vi "Access insert values.vi"(5 "是否创建唯一键":bool, 6 "Password":string, 7 "data":variant[](array[variant]), 8 "error in (no error)":errorcluster, 9 "columns外部输入":T1, 10 "database":string="database1.mdb", 11 "table":string) -> (0 "error out":errorcluster)   [LabVIEW 2016, in "Access Lib.lvlib"]
uses:
  Access Lib.lvlib
  <vilib>/addons/database/Auxilliary.llb/DB Tools Transaction.ctl
  <vilib>/addons/database/Auxilliary.llb/DB Tools Isolation Level.ctl
  <vilib>/addons/database/Auxilliary.llb/DB Tools Column Info.ctl
  <vilib>/addons/database/Auxilliary.llb/DB Tools DataTypes.ctl
  <vilib>/addons/database/Auxilliary.llb/DB Tools Parameter Info.ctl
  <vilib>/addons/database/Auxilliary.llb/DB Tools Parameter Dir.ctl
  <vilib>/addons/database/Connection.llb/DB Tools Open Connec (String).vi
  <vilib>/addons/database/Connection.llb/Conn Transaction.vi
  <vilib>/addons/database/Connection.llb/Conn Execute.vi
  <vilib>/addons/database/Recordset.llb/Rec Destroy - Connection.vi
  <vilib>/addons/database/Command.llb/Cmd Set Parameter Value (C).vi
  <vilib>/addons/database/Command.llb/Cmd Execute.vi
  <vilib>/addons/database/Recordset.llb/Rec Destroy - Command.vi
  <vilib>/addons/database/Command.llb/Cmd Delete.vi
  <vilib>/addons/database/NI_Database_API.lvlib
  <vilib>/Utility/VariantDataType/VariantType.lvlib
panel:
  out "当前数据时间":timestamp
  out "当前测量模式":string
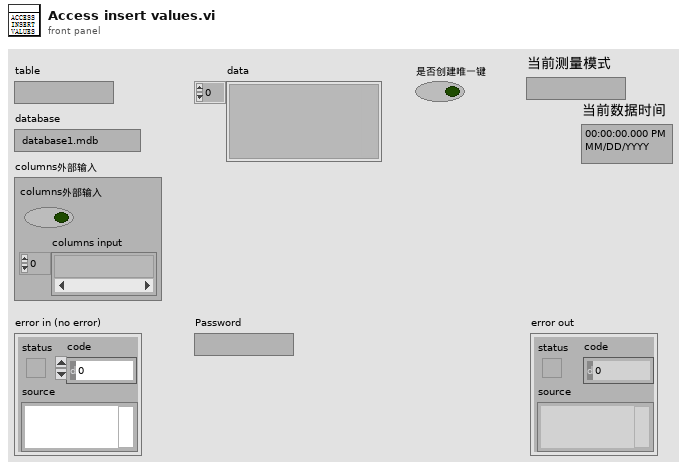
[diagram p1: front panel]
types:
  T1 = cluster{"columns外部输入":bool, "columns input":string[]}
  T2 = typedef "NI_Database_API.lvlib/DB Tools Isolation Level.ctl" = enum16{"chaos", "read uncommitted", "read committed", "repeatable read", "serializable"}
  T3 = typedef "NI_Database_API.lvlib/DB Tools Transaction.ctl" = enum16{"begin", "commit", "rollback"}
  T4 = typedef "NI_Database_API.lvlib/DB Tools Column Info.ctl" = cluster{"column name":string, "data type":T5, "size":i32, "allow null?":bool}
  T5 = typedef "NI_Database_API.lvlib/DB Tools DataTypes.ctl" = enum16{"String", "Long (I32)", "Single (SGL)", "Double (DBL)", "Date/Time", "Binary"}
  T6 = typedef "VariantType.lvlib/Type.ctl" = enum8{"Invalid Type", "Void", "I8", "I16", "I32", "I64", "U8", "U16", "U32", "U64", "Single Float", "Double Float", "Extended Float", "Single Complex", "Double Complex", "Extended Complex", "Enum U8", "Enum U16", "Enum U32", "Enum U64", "Single Float With Unit", "Double Float With Unit", "Extended Float With Unit", "Single Complex with Unit", "Double Complex with Unit", "Extended Complex with Unit", "Boolean", "String", "Path", "Picture", "Tag", "Array", "Cluster", "Variant", "LV Variant", "Waveform", "Timestamp", "Digital Waveform", "Digital Data", "ExpressData", "Refnum", "External Data", "VI", "Poly VI", "LabVIEW Class Instance", "Fixed Point"}
  T7 = typedef "NI_Database_API.lvlib/Conn ObjectReference.ctl" = refnum<k1>
  T8 = typedef "NI_Database_API.lvlib/DB Tools Parameter Info.ctl" = cluster{"parameter name":string, "type":T5, "direction":T9, "value":variant}
  T9 = typedef "NI_Database_API.lvlib/DB Tools Parameter Dir.ctl" = enum32{"Input", "Output", "Input/Output", "Return Value"}
  T10 = typedef "NI_Database_API.lvlib/Rec ObjectReference.ctl" = refnum<k1>
  T11 = typedef "LVDateTimeRec.ctl" = cluster{"秒数的小数部分":dbl, "秒":i32, "分":i32, "时":i32, "日":i32, "月":i32, "年":i32, "天数（周）":i32, "天数（年）":i32, "DST":i32}
  T12 = typedef "NI_Database_API.lvlib/Cmd ObjectReference.ctl" = refnum<k1>
  T13 = typedef "NI_Database_API.lvlib/Cmd-Rec Object Reference.ctl" = refnum<k1>
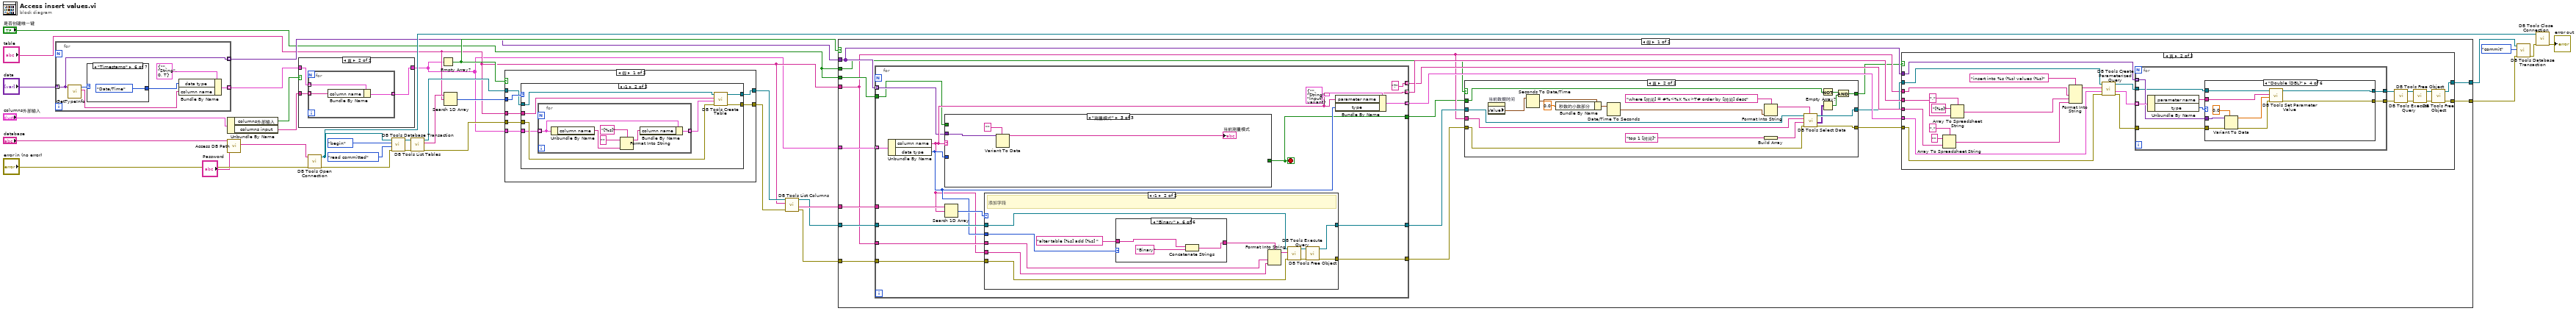
[diagram p0: block diagram]
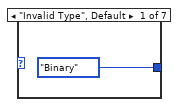
[diagram p3: hidden frame]
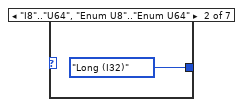
[diagram p4: hidden frame]
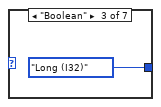
[diagram p5: hidden frame]
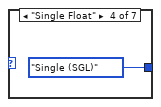
[diagram p6: hidden frame]
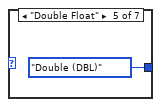
[diagram p7: hidden frame]
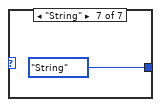
[diagram p8: hidden frame]
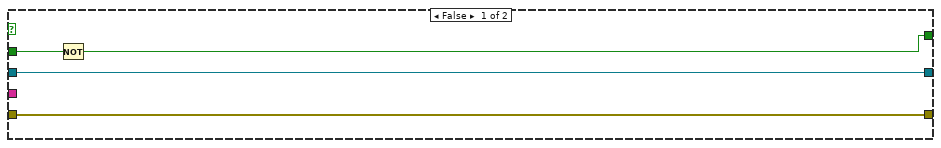
[diagram p11: hidden frame]
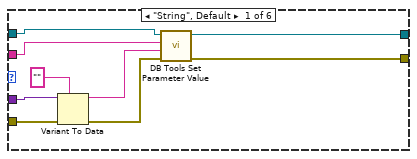
[diagram p13: hidden frame]
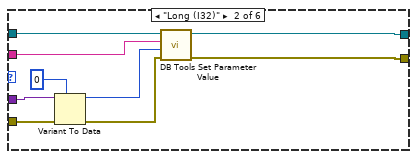
[diagram p14: hidden frame]
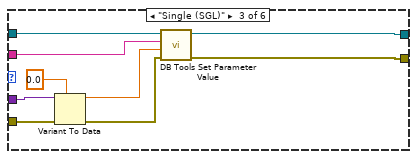
[diagram p15: hidden frame]
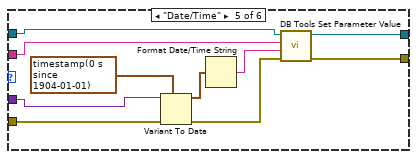
[diagram p16: hidden frame]
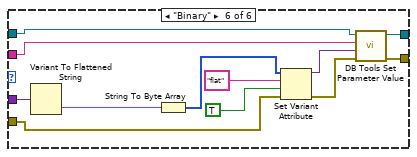
[diagram p17: hidden frame]
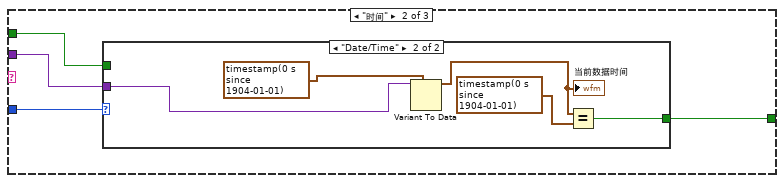
[diagram p19: hidden frame]
diagram:
  n1 = for {
    tunnel: [w35] -> w12 mode=indexing
    tunnel: [w37] -> w9 mode=indexing
    tunnel: "data" -> [w35] mode=indexing
    n2 = call <vilib>:"GetTypeInfo.vi"("Variant"=w35) -> ("Name"=w36:string, "Type Enum"=w39:T6)  [unwired: 6 in, 3 out]
    n3 = case shown="\"Timestamp\"" w39 {
      tunnel: [DB_Tools_DataTypes."Binary" ("data type") DB_Tools_DataTypes."Long (I32)" ("data type") DB_Tools_DataTypes."Long (I32)" ("data type") DB_Tools_DataTypes."Single (SGL)" ("data type") DB_Tools_DataTypes."Double (DBL)" ("data type") DB_Tools_DataTypes."Date/Time" ("data type") DB_Tools_DataTypes."String" ("data type")] -> w38
      frame "Invalid Type", Default {
      }
      frame "I8".."U64", "Enum U8".."Enum U64" {
      }
      frame "Boolean" {
      }
      frame "Single Float" {
      }
      frame "Double Float" {
      }
      frame "Timestamp" {
      }
      frame "String" {
      }
    }
    n4 = Bundle By Name(cluster=T4 {"column name"="", "data type"=enum."String", "size"=0, "allow null?"=TRUE} ("column information"), "data type"=w38, "column name"=w36) -> (w37:T4)
  }
  n5 = Unbundle By Name("columns外部输入") -> ("columns外部输入"=w7:bool, "columns input"=w8:string[])
  n6 = call "Access DB Path.vi"("Password"="Password", "database"="database") -> ("Connection information"=w5:string)  [unwired: 8 in, 1 out]
  n7 = case shown="真" w7 {
    tunnel: w9 -> [w48 w51]
    tunnel: [w48 w50] -> w6
    tunnel: w8 -> [_ w49]
    frame False {
    }
    frame True {
      n8 = for {
        tunnel: w51 -> [w54] mode=indexing
        tunnel: [w53] -> w50 mode=indexing
        tunnel: w49 -> [w52] mode=indexing
        n9 = Bundle By Name(cluster=w54, "column name"=w52) -> (w53:T4)
      }
    }
  }
  n10 = call-poly <vilib>:"DB Tools Open Connection.vi"("error in (no error)"="error in (no error)", "connection information"=w5) -> ("error out"=w19:errorcluster, "connection reference"=w16:T7)  [unwired: 6 in]
  n11 = call-poly <vilib>:"DB Tools Database Transaction.vi"("error in (no error)"=w19, "isolation level (chaos)"=DB_Tools_Isolation_Level."read committed", "operation (begin)"=DB_Tools_Transaction."begin", "connection reference"=w16) -> ("error out"=w18:errorcluster, "connection reference out"=w20:T7)  [unwired: 2 in]
  n12 = call <vilib>:"DB Tools List Tables.vi"("error in (no error)"=w18, "connection reference"=w20) -> ("error out"=w27:errorcluster, "tables"=w29:string[], "connection reference out"=w17:T7)  [unwired: 3 in]
  n13 = Empty Array?(array=w6) -> (empty?=w14:bool)
  n14 = Search 1D Array(1D array=w29, element="table") -> (index of element=w28:i32)  [unwired: 1 in]
  n15 = case shown="假" w14 {
    tunnel: w28 -> [w61 _]
    tunnel: w27 -> [w60 w77]
    tunnel: [w59 w78] -> w25
    tunnel: [w58 w77] -> w24
    tunnel: w17 -> [w57 w78]
    tunnel: "table" -> [w56 _]
    tunnel: w6 -> [w55 _]
    frame False {
      n16 = case shown="-1" w61 {
        tunnel: w57 -> [w63 w70]
        tunnel: w60 -> [w62 w69]
        tunnel: w56 -> [_ w68]
        tunnel: w55 -> [_ w65]
        tunnel: [w63 w67] -> w59
        tunnel: [w62 w66] -> w58
        frame 0, Default {
        }
        frame -1 {
          n17 = for {
            tunnel: w65 -> [w72] mode=indexing
            tunnel: [w71] -> w64 mode=indexing
            n18 = Unbundle By Name(w72) -> ("column name"=w76:string)
            n19 = Format Into String(format string="[%s]" ("格式字符串"), initial string="" ("初始字符串"), w76) -> (resulting string=w73:string)  [unwired: 1 in, 1 out]
            n20 = Bundle By Name(cluster=w72, "column name"=w73) -> (w71:T4)
          }
          n21 = call <vilib>:"DB Tools Create Table.vi"("error in (no error)"=w69, "column information"=w64, "table"=w68, "connection reference"=w70) -> ("error out"=w66:errorcluster, "connection reference out"=w67:T7)  [unwired: 4 in]
        }
      }
    }
    frame True {
    }
  }
  n22 = call <vilib>:"DB Tools List Columns.vi"("error in (no error)"=w24, "table"="table", "connection reference"=w25) -> ("error out"=w3:errorcluster, "columns"=w26:string[], "connection reference out"=w4:T7)  [unwired: 1 in, 1 out]
  n23 = case shown="假" w14 {
    tunnel: w26 -> [w97 _]
    tunnel: w3 -> [w96 w275]
    tunnel: [w92 w276] -> w22
    tunnel: [w91 w275] -> w21
    tunnel: w12 -> [w88 _]
    tunnel: w4 -> [w90 w276]
    tunnel: "table" -> [w82 _]
    tunnel: w6 -> [w89 _]
    tunnel: "是否创建唯一键" -> [w87 _]
    tunnel: "是否创建唯一键" -> [w80 _]
    frame False {
      n24 = for {
        tunnel: w90 -> [w228]
        tunnel: w97 -> [w230]
        tunnel: w96 -> [w227]
        tunnel: [w226] -> w84
        tunnel: w82 -> [w225]
        tunnel: w89 -> [w224] mode=indexing
        tunnel: [w222] -> w95 mode=indexing
        tunnel: [w218] -> w94 mode=indexing
        tunnel: ["?"] -> w93 mode=indexing
        tunnel: [w220] -> w86
        tunnel: w88 -> [w217] mode=indexing
        tunnel: [w216] -> w81
        tunnel: w87 -> [w215]
        stop <- w216 stop-if-true
        n25 = Unbundle By Name(w224) -> ("column name"=w218:string, "data type"=w219:T5)
        n26 = case shown="\"测量模式\"" w218 {
          tunnel: w219 -> [_ w234 _]
          tunnel: w217 -> [_ w233 w242]
          tunnel: [_ w232 _] -> w216
          tunnel: w215 -> [_ w231 _]
          frame "假", Default {
          }
          frame "时间" {
            n27 = case shown="\"Date/Time\"" w234 {
              tunnel: w233 -> [_ w239]
              tunnel: [_ w235] -> w232
              tunnel: w231 -> [_ _]
              frame "String", Default {
              }
              frame "Date/Time" {
                n28 = Variant To Data(type=timestamp(0 s since 1904-01-01) ("时间标识"), Variant=w239) -> (data=w237:timestamp)  [unwired: 1 in, 1 out]
                "当前数据时间" <- w237
                n29 = Equal?(x=w237, y=timestamp(0 s since 1904-01-01) ("时间标识")) -> (x = y?=w235:bool)
              }
            }
          }
          frame "测量模式" {
            n30 = Variant To Data(type="", Variant=w242) -> (data=→"当前测量模式":string)  [unwired: 1 in, 1 out]
          }
        }
        n31 = Search 1D Array(1D array=w230, element=w218) -> (index of element=w229:i32)  [unwired: 1 in]
        n32 = case shown="-1" w229 {
          tunnel: [w244 w253] -> w226
          tunnel: w228 -> [w243 w252]
          tunnel: w218 -> [_ w251]
          tunnel: w227 -> [w244 w250]
          tunnel: w225 -> [_ w249]
          tunnel: w219 -> [_ w247]
          tunnel: [w243 w245] -> w220
          frame 0, Default {
          }
          frame -1 {
            # "添加字段"
            n33 = case shown="\"Binary\"" w247 {
              tunnel: "alter table [%s] add [%s] " -> [w259 w262 w265 w268 w271 w274]
              tunnel: [w258 w261 w264 w267 w270 w273] -> w246
              frame "String", Default {
                n34 = Concatenate Strings(w259, "String" ("字符串")) -> (w258:string)
              }
              frame "Long (I32)" {
                n35 = Concatenate Strings(w262, "Long" ("字符串")) -> (w261:string)
              }
              frame "Single (SGL)" {
                n36 = Concatenate Strings(w265, "Single" ("字符串")) -> (w264:string)
              }
              frame "Double (DBL)" {
                n37 = Concatenate Strings(w268, "Double" ("字符串")) -> (w267:string)
              }
              frame "Date/Time" {
                n38 = Concatenate Strings(w271, "TimeStamp" ("字符串")) -> (w270:string)
              }
              frame "Binary" {
                n39 = Concatenate Strings(w274, "Binary" ("字符串")) -> (w273:string)
              }
            }
            n40 = Format Into String(format string=w246, w249, w251) -> (resulting string=w254:string)  [unwired: 2 in, 1 out]
            n41 = call-poly <vilib>:"DB Tools Execute Query.vi"("error in (no error)"=w250, "SQL query"=w254, "connection reference"=w252) -> ("error out"=w255:errorcluster, "recordset reference"=w256:T10)  [unwired: 5 in]
            n42 = call-poly <vilib>:"DB Tools Free Object.vi"("error in (no error)"=w255, "recordset reference"=w256) -> ("error out"=w253:errorcluster, "connection reference"=w245:T7)  [unwired: 8 in]
          }
        }
        n43 = Bundle By Name(cluster=T8 {"parameter name"="", "type"=enum."String", "direction"=enum."Input", "value"=variant} ("parameter information"), "parameter name"=w218, "type"=w219) -> (w222:T8)
      }
      n44 = case shown="真" w80 {
        tunnel: w86 -> [w101 w118]
        tunnel: [w101 w117] -> w85
        tunnel: w84 -> [w100 w116]
        tunnel: [w100 w115] -> w83
        tunnel: w82 -> [_ w114]
        tunnel: w81 -> [w99 w103]
        tunnel: [w98 w105] -> w79
        frame False {
          n45 = Not(x=w99) -> (.not. x?=w98:bool)
        }
        frame True {
          n46 = property on="当前数据时间" class="AbsTime (严格)"() -> ("Value"=w111:timestamp)  [unwired: 2 in, 2 out]
          n47 = Seconds To Date/Time(time stamp (now)=w111) -> (date time rec=w110:T11)  [unwired: 1 in]
          n48 = Bundle By Name(cluster=w110, "秒数的小数部分"=0.0) -> (w107:T11)
          n49 = Date/Time To Seconds(2:w107) -> (0:w108:timestamp)  [unwired: 1 in]
          n50 = Format Into String(format string="where [时间] = #%<%X %x>T# order by [时间] desc" ("condition"), w108) -> (resulting string=w113:string)  [unwired: 2 in, 1 out]
          n51 = Build Array("top 1 [时间]") -> (w120:string[])
          n52 = call <vilib>:"DB Tools Select Data.vi"("condition"=w113, "error in (no error)"=w116, "columns"=w120, "table"=w114, "connection reference"=w118) -> ("error out"=w115:errorcluster, "data"=w106:variant[][], "connection reference out"=w117:T7)  [unwired: 1 in]
          n53 = Not(x=w103) -> (.not. x?=w102:bool)
          n54 = Empty Array?(array=w106) -> (empty?=w104:bool)
          n55 = And(x=w102, y=w104) -> (x .and. y?=w105:bool)
        }
      }
      n56 = case shown="真" w79 {
        tunnel: w95 -> [_ w148]
        tunnel: w94 -> [_ w142]
        tunnel: w93 -> [_ w140]
        tunnel: [w122 w130] -> w92
        tunnel: [w121 w129] -> w91
        tunnel: w85 -> [w122 w127]
        tunnel: w83 -> [w121 w125]
        tunnel: w82 -> [_ w124]
        tunnel: w88 -> [_ w123]
        frame False {
        }
        frame True {
          n57 = Array To Spreadsheet String(delimiter (Tab)="," ("分隔符(Tab)"), array=w140, 3:"" ("格式字符串")) -> (spreadsheet string=w139:string)
          n58 = Array To Spreadsheet String(delimiter (Tab)="," ("分隔符(Tab)"), array=w142, 3:"[%s]" ("格式字符串")) -> (spreadsheet string=w141:string)
          n59 = Format Into String(format string="insert into %s (%s) values (%s)" ("格式字符串"), w124, w141, w139) -> (resulting string=w138:string)  [unwired: 2 in, 1 out]
          n60 = call <vilib>:"DB Tools Create Parameterized Query.vi"("error in (no error)"=w125, "parameters"=w148, "SQL query"=w138, "connection reference"=w127) -> ("error out"=w137:errorcluster, "parameters out"=w136:T8[], "command reference"=w128:T12)  [unwired: 3 in]
          n61 = for {
            tunnel: w128 -> [w153]
            tunnel: w137 -> [w151]
            tunnel: w136 -> [w156] mode=indexing
            tunnel: w123 -> [w154] mode=indexing
            tunnel: [w150] -> w126
            tunnel: [w149] -> w135
            n62 = Unbundle By Name(w156) -> ("parameter name"=w152:string, "type"=w155:T5)
            n63 = case shown="\"Double (DBL)\"" w155 {
              tunnel: w154 -> [w160 w168 w175 w185 w202 w206]
              tunnel: w153 -> [w163 w172 w179 w189 w200 w214]
              tunnel: w152 -> [w162 w171 w178 w184 w195 w213]
              tunnel: w151 -> [w157 w166 w176 w186 w198 w205]
              tunnel: [w159 w170 w180 w188 w197 w212] -> w150
              tunnel: [w158 w169 w177 w187 w196 w211] -> w149
              frame "String", Default {
                n64 = Variant To Data(error in=w157, type="", Variant=w160) -> (data=w161:string, error out=w165:errorcluster)
                n65 = call-poly <vilib>:"DB Tools Set Parameter Value.vi"("error in (no error)"=w165, "value"=w161, "parameter index"=w162, "command reference"=w163) -> ("error out"=w158:errorcluster, "command reference out"=w159:T12)  [unwired: 4 in]
              }
              frame "Long (I32)" {
                n66 = Variant To Data(error in=w166, type=0, Variant=w168) -> (data=w173:i32, error out=w174:errorcluster)
                n67 = call-poly <vilib>:"DB Tools Set Parameter Value.vi"("error in (no error)"=w174, "value"=w173, "parameter index"=w171, "command reference"=w172) -> ("error out"=w169:errorcluster, "command reference out"=w170:T12)  [unwired: 4 in]
              }
              frame "Single (SGL)" {
                n68 = Variant To Data(error in=w176, type=sgl 0.0, Variant=w175) -> (data=w182:sgl, error out=w183:errorcluster)
                n69 = call-poly <vilib>:"DB Tools Set Parameter Value.vi"("error in (no error)"=w183, "value"=w182, "parameter index"=w178, "command reference"=w179) -> ("error out"=w177:errorcluster, "command reference out"=w180:T12)  [unwired: 4 in]
              }
              frame "Double (DBL)" {
                n70 = Variant To Data(error in=w186, type=0.0, Variant=w185) -> (data=w191:dbl, error out=w192:errorcluster)
                n71 = call-poly <vilib>:"DB Tools Set Parameter Value.vi"("error in (no error)"=w192, "value"=w191, "parameter index"=w184, "command reference"=w189) -> ("error out"=w187:errorcluster, "command reference out"=w188:T12)  [unwired: 4 in]
              }
              frame "Date/Time" {
                n72 = Variant To Data(error in=w198, type=timestamp(0 s since 1904-01-01) ("时间标识"), Variant=w202) -> (data=w194:timestamp, error out=w199:errorcluster)
                n73 = Format Date/Time String(seconds (now)=w194) -> (date/time string=w193:string)  [unwired: 2 in]
                n74 = call-poly <vilib>:"DB Tools Set Parameter Value.vi"("error in (no error)"=w199, "value"=w193, "parameter index"=w195, "command reference"=w200) -> ("error out"=w196:errorcluster, "command reference out"=w197:T12)  [unwired: 4 in]
              }
              frame "Binary" {
                n75 = Variant To Flattened String(Variant=w206) -> (data string=w207:string)  [unwired: 1 out]
                n76 = String To Byte Array(string=w207) -> (unsigned byte array=w210:u8[])
                n77 = Set Variant Attribute(Variant=w210, name="flat", value=TRUE, error in=w205) -> (Variant out=w203:variant, error out=w204:errorcluster)  [unwired: 1 out]
                n78 = call-poly <vilib>:"DB Tools Set Parameter Value.vi"("error in (no error)"=w204, "value"=w203, "parameter index"=w213, "command reference"=w214) -> ("error out"=w211:errorcluster, "command reference out"=w212:T12)  [unwired: 4 in]
              }
            }
          }
          n79 = call-poly <vilib>:"DB Tools Execute Query.vi"("error in (no error)"=w135, "command reference"=w126) -> ("error out"=w133:errorcluster, "command-recordset reference"=w134:T13)  [unwired: 6 in]
          n80 = call-poly <vilib>:"DB Tools Free Object.vi"("error in (no error)"=w133, "command-recordset reference"=w134) -> ("error out"=w131:errorcluster, "command reference"=w132:T12)  [unwired: 8 in]
          n81 = call-poly <vilib>:"DB Tools Free Object.vi"("error in (no error)"=w131, "command reference"=w132) -> ("error out"=w129:errorcluster, "connection reference"=w130:T7)  [unwired: 8 in]
        }
      }
    }
    frame True {
    }
  }
  n82 = call-poly <vilib>:"DB Tools Database Transaction.vi"("error in (no error)"=w21, "operation (begin)"=DB_Tools_Transaction."commit", "connection reference"=w22) -> ("error out"=w23:errorcluster)  [unwired: 3 in, 1 out]
  n83 = call <vilib>:"DB Tools Close Connection.vi"("error in (no error)"=w23, "connection reference"=w16) -> ("error out"=→"error out":errorcluster)  [unwired: 5 in]
